vi "Update Dynamic VI DLL Methods.vi"(4 "MethodName":string, 6 "DLL Path":path, 8 "error in":errorcluster, 9 "Custom Device Name":string, 10 "NameSpace":string, 11 "VI path":path) -> (0 "error out":errorcluster)   [LabVIEW 2026, in "NIVS_CDEW_MetaDataObj.lvclass"]
uses:
  NIVS_CDEW_MetaDataObj.lvclass
  NIVS_CDEW_MetaDataObj.lvclass/NIVS_CDEW_MetaDataObj.ctl
  <vilib>/Utility/traverseref.llb/TRef TravTarget.ctl
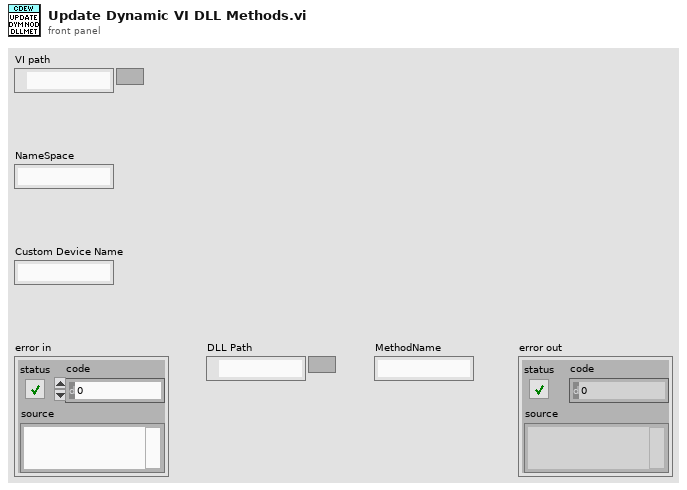
[diagram p1: front panel]
types:
  T1 = typedef "TRef TravTarget.ctl" = enum16{"FP", "BD", "Other"}
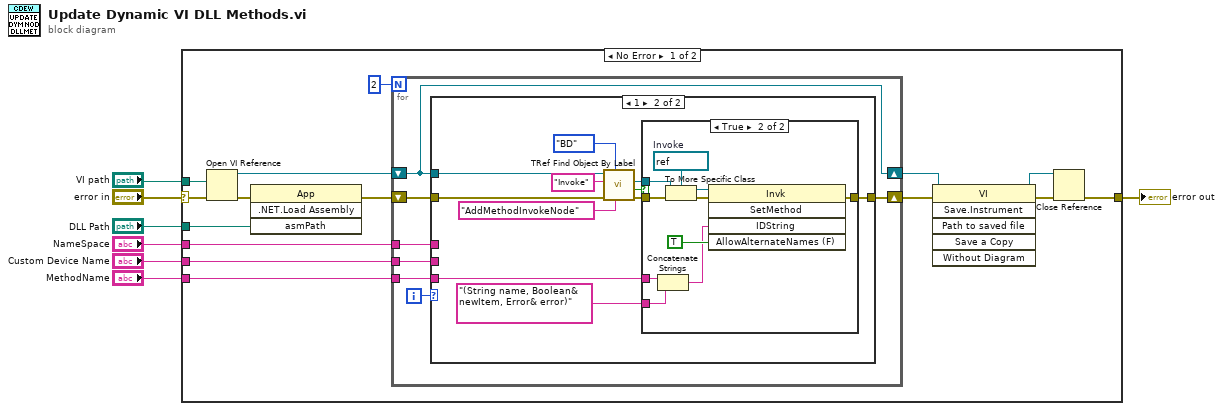
[diagram p0: block diagram]
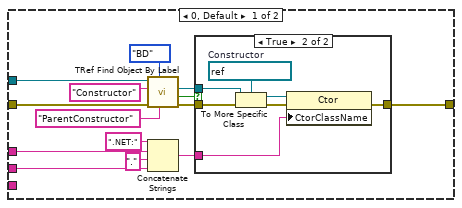
[diagram p2: hidden frame]
diagram:
  n1 = case shown="No Error" "error in" {
    selector: "error in" -> [w18 w74]
    tunnel: "VI path" -> [w22 _]
    tunnel: "DLL Path" -> [w21 _]
    tunnel: "NameSpace" -> [w16 _]
    tunnel: "Custom Device Name" -> [w15 _]
    tunnel: "MethodName" -> [w13 _]
    tunnel: [w12 w74] -> w1
    frame No Error {
      n2 = Open VI Reference(vi path=w22, error in (no error)=w18) -> (vi reference=w19:refnum<vi>, error out=w20:errorcluster)  [unwired: 4 in]
      n3 = invoke class="App" method=".NET.Load Assembly"(error in=w20, "asmPath"=w21) -> (error out=w17:errorcluster)  [unwired: 2 in, 3 out]
      n4 = for {
        N: 2 -> [_]
        tunnel: w16 -> [w27]
        tunnel: w15 -> [w26]
        shift-right: [w23] -> w9
        shift-left: w19 -> [w23]
        shift-right: [w29] -> w11
        shift-left: w17 -> [w28]
        tunnel: w13 -> [w24]
        i -> [w25]
        n5 = case shown="1" w25 {
          tunnel: w23 -> [w43 w62]
          tunnel: [w35 w56] -> w29
          tunnel: w28 -> [w36 w54]
          tunnel: w27 -> [w33 _]
          tunnel: w26 -> [w31 _]
          tunnel: w24 -> [_ w53]
          frame 0, Default {
            n6 = call <vilib>:"TRef Find Object By Label.vi"("Label"="ParentConstructor", "Traverse Target"=TRef_TravTarget."BD", "error in (no error)"=w36, "Class Name"="Constructor", "VI Ref"=w43) -> ("error out"=w38:errorcluster, "Found?"=w40:bool, "Found Obj Ref"=w39:refnum<vi>)  [unwired: 3 in, 1 out]
            n7 = Concatenate Strings(".NET:", w33, ".", w31) -> (w30:string)
            n8 = case shown="True" w40 {
              tunnel: w39 -> [_ w51]
              tunnel: w38 -> [w44 w50]
              tunnel: [w44 w46] -> w35
              tunnel: w30 -> [_ w45]
              frame False {
              }
              frame True {
                w49 = refnum<vi> refnum  # Constructor
                n9 = To More Specific Class(target class=w49, reference=w51, error in=w50) -> (specific class reference=w47:refnum<vi>, error out=w48:errorcluster)
                n10 = property class="Ctor"(reference=w47, error in=w48, "CtorClassName"=w45) -> (error out=w46:errorcluster)  [unwired: 1 out]
              }
            }
          }
          frame 1 {
            n11 = call <vilib>:"TRef Find Object By Label.vi"("Label"="AddMethodInvokeNode", "Traverse Target"=TRef_TravTarget."BD", "error in (no error)"=w54, "Class Name"="Invoke", "VI Ref"=w62) -> ("error out"=w57:errorcluster, "Found?"=w59:bool, "Found Obj Ref"=w58:refnum<vi>)  [unwired: 3 in, 1 out]
            n12 = case shown="True" w59 {
              tunnel: w58 -> [_ w73]
              tunnel: w57 -> [w63 w72]
              tunnel: [w63 w68] -> w56
              tunnel: w53 -> [_ w66]
              tunnel: "(String name, Boolean& newItem, Error& error)" ("Label") -> [_ w65]
              frame False {
              }
              frame True {
                w71 = refnum<vi> refnum  # Invoke
                n13 = Concatenate Strings(w66, w65) -> (w64:string)
                n14 = To More Specific Class(target class=w71, reference=w73, error in=w72) -> (specific class reference=w70:refnum<vi>, error out=w69:errorcluster)
                n15 = invoke class="Invk" method="SetMethod"(reference=w70, error in=w69, "IDString"=w64, "AllowAlternateNames (F)"=TRUE ("Allow Alternate Names? (F)")) -> (error out=w68:errorcluster)  [unwired: 1 in, 4 out]
              }
            }
          }
        }
      }
      n16 = invoke class="VI" method="Save.Instrument"(reference=w9, error in=w11) -> (reference out=w8:refnum<vi>, error out=w10:errorcluster)  [unwired: 4 in, 4 out]
      n17 = Close Reference(reference=w8, error in (no error)=w10) -> (error out=w12:errorcluster)
    }
    frame Error {
    }
  }
  "error out" <- w1
